vi "VisOpenQueue.vi"(8 "Error Array In":errorcluster[](array[cluster]), 11 "QueueName":string) -> (0 "Error Array Out":errorcluster[](array[cluster]), 3 "queue out":refnum<queue>)   [LabVIEW 2018, in "Visualization.lvlib" / "VisualizeBase.lvclass"]
doc: "This VI opens a queue."
uses:
  VisualizeBase/VisualizeBase_class/VisualizeBase.lvclass
  <userlib>/NIST/NISTErrorLib/NISTErrorLib.lvlib
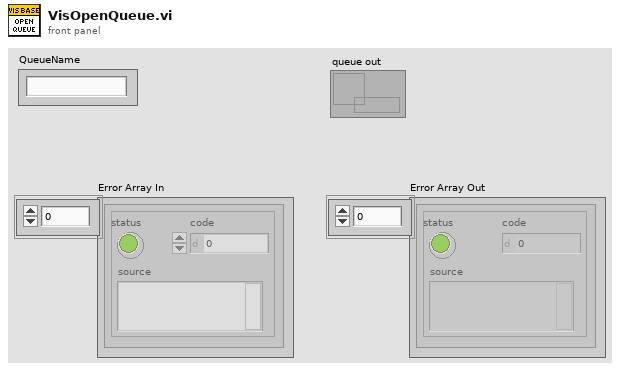
[diagram p1: front panel]
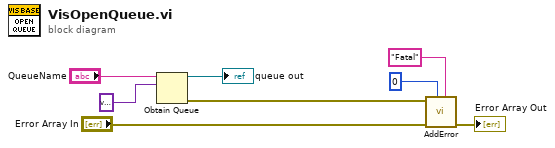
[diagram p0: block diagram]
diagram:
  n1 = Obtain Queue(name (unnamed)="QueueName", element data type=variant) -> (queue out=→"queue out":refnum<queue>, error out=w2:errorcluster)  [unwired: 3 in, 1 out]
  n2 = call <userlib>:"AddError.vi"("Severity"="Fatal", "Priority"=u8 0, "ErrorArray In"="Error Array In", "error in (no error)"=w2) -> ("ErrorArray Out"=→"Error Array Out":errorcluster[])  [unwired: 6 in, 1 out]
